vi "Initialize Manager Tab by Reference.vi"(8 "error in (no error)":errorcluster, 11 "CIF Manager UI Tab":refnum<vi>) -> (0 "error out":errorcluster)   [LabVIEW 2021, in "CIF_Manager_UI.lvclass"]
uses:
  CIF_Manager_UI.lvclass
  Typedef/CIF_Manager_UI_Tab.ctl
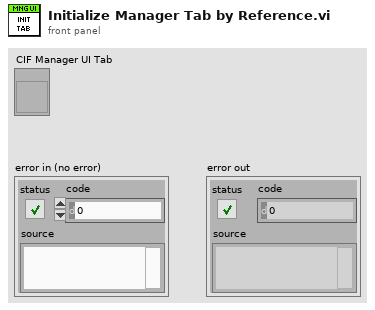
[diagram p1: front panel]
types:
  T1 = typedef "CIF_Manager_UI.lvclass/CIF_Manager_UI_Tab.ctl" = enum32{"System Management", "Channels", "Monitoring and Errors", "Plugin UI"}
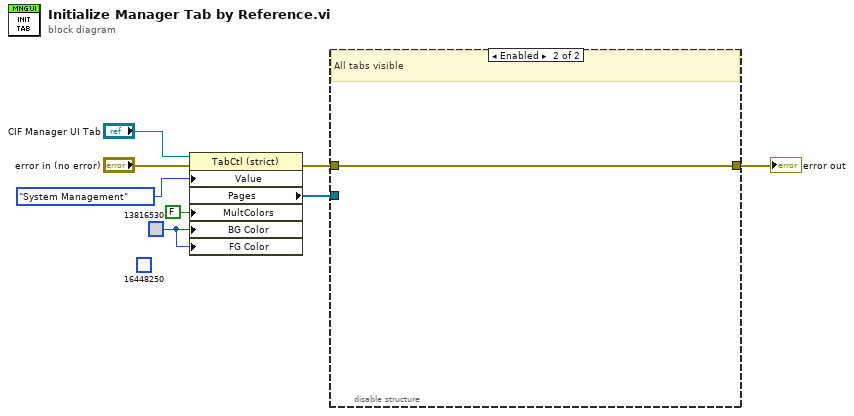
[diagram p0: block diagram]
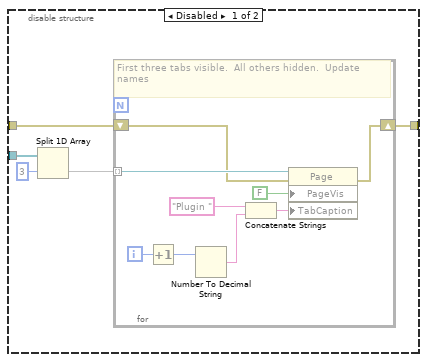
[diagram p2: hidden frame]
diagram:
  (unwired) u32 16448250 ("Colors:FG Color")
  w2 = u32 13816530 ("Colors:BG Color")
  n1 = property on="Property Node" class="TabCtl (strict)"(reference="CIF Manager UI Tab", error in="error in (no error)", "Value"=CIF_Manager_UI_Tab."System Management", "MultColors"=FALSE ("Allow Multiple Colors"), "BG Color"=w2, "FG Color"=w2) -> (error out=w6:errorcluster, "Pages"=w4:refnum<vi>[])  [unwired: 1 out]
  n2 = disable-structure shown="Enabled" {
    disable-tunnel: w6 -> [w13 w23]
    disable-tunnel: [w12 w23] -> w5
    disable-tunnel: w4 -> [w11 _]
    frame Disabled {
      n3 = Split 1D Array(array=w11, index=3) -> (second subarray=w9:refnum<vi>[])  [unwired: 1 out]
      n4 = for {
        tunnel: w9 -> [w22] mode=indexing
        shift-right: [w20] -> w12
        shift-left: w13 -> [w21]
        i -> [w18]
        # "First three tabs visible.  All others hidden.  Update names"
        n5 = Increment(x=w18) -> (x+1=w17:i32)
        n6 = Number To Decimal String(number=w17) -> (decimal integer string=w16:string)  [unwired: 1 in]
        n7 = Concatenate Strings("Plugin " ("string"), w16) -> (w14:string)
        n8 = property on="Property Node" class="Page"(reference=w22, error in=w21, "PageVis"=FALSE ("Page Visible"), "TabCaption"=w14) -> (error out=w20:errorcluster)  [unwired: 1 out]
      }
    }
    frame Enabled {
      # "All tabs visible"
    }
  }
  "error out" <- w5
